vi "OdometrySubscriber.vi"() -> ()   [LabVIEW 2014]
doc: "Reads in the odometry from the Turtlebot"
uses:
  <vilib>/Tufts CEEO ROS for LabVIEW Software/ROS/Code/Console/Servers/ServerSubs/TopicDef.ctl
  <vilib>/Tufts CEEO ROS for LabVIEW Software/ROS/Code/SubVIs/_ROSDirection.ctl
panel:
  out "Odom Error Out":errorcluster
  in  "Update Time (ms)":u32
  in  "Clear Plot":bool
  out "2D Pose":cluster{"x":dbl, "y":dbl}
  out "Position Plot":cluster{"X":dbl, "Y":dbl}[](graph)
  out "Husky EKF Odometry":T1
  in  "Stop Subscribing":bool
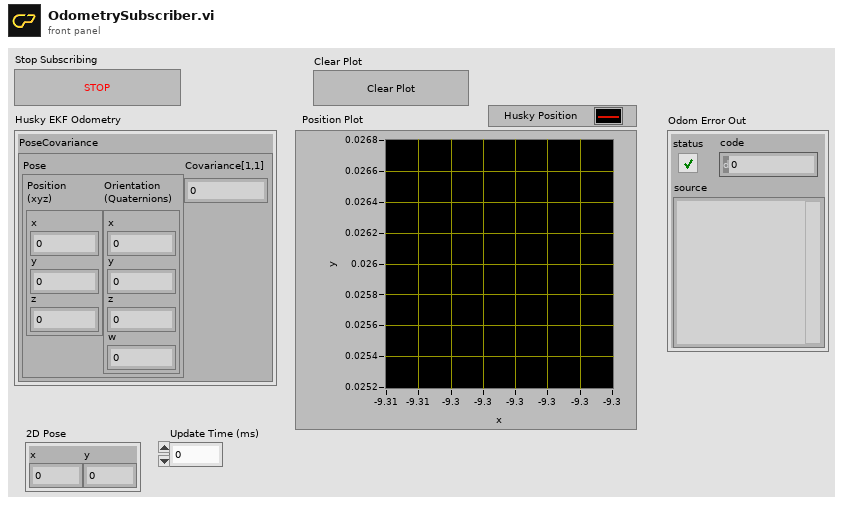
[diagram p1: front panel]
types:
  T1 = cluster{"PoseCovariance":cluster{"Pose":cluster{"Position\n(xyz)":cluster{"x":dbl, "y":dbl, "z":dbl}, "Orientation\n(Quaternions)":cluster{"x":dbl, "y":dbl, "z":dbl, "w":dbl}}, "Covariance[1,1]":dbl}}
  T2 = typedef "TopicDef.ctl" = cluster{"Topic":string, "Type":string, "Action":T3, "Update (ms)":u16, "queue size":u16}
  T3 = typedef "_ROSDirection.ctl" = enum16{"Node", "Publisher", "Subscriber", "ServiceClient", "ServiceProvider"}
  T4 = typedef "_ROSControl.ctl" = cluster{"topic port":u16, "Node":string, "topic":string, "type":string, "node port":u16, "error ":errorcluster, "Direction":T3, "Update (ms)":u16, "FIFO size":u16}
  T5 = cluster{"PoseCovariance":cluster{"Pose":cluster{"Point":cluster{"x":dbl, "y":dbl, "z":dbl}, "Quaternion":cluster{"x":dbl, "y":dbl, "z":dbl, "w":dbl}}, "Covariance":dbl}}
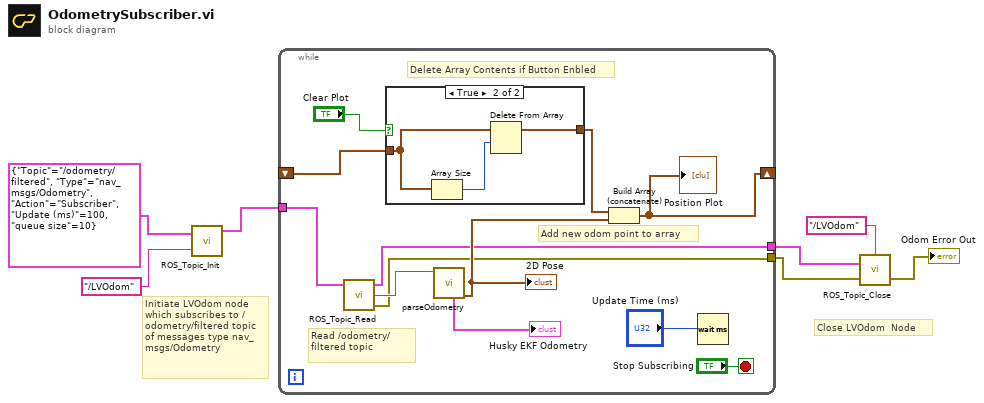
[diagram p0: block diagram]
diagram:
  # "Initiate LVOdom node which subscribes to /odometry/filtered topic of messages type nav_msgs/Odometry"
  # "Close LVOdom  Node"
  n1 = call <vilib>:"ROS_Topic_Init.vi"("Definitions"=T2 {"Topic"="/odometry/filtered", "Type"="nav_msgs/Odometry", "Action"=enum."Subscriber", "Update (ms)"=100, "queue size"=10}, "node"="/LVOdom") -> ("ROS out"=w5:T4)  [unwired: 1 in, 1 out]
  n2 = while {
    shift-right: [w13] -> _
    shift-left: _ -> [w14]
    tunnel: w5 -> [w16]
    tunnel: [w9] -> w2
    tunnel: [w8] -> w1
    stop <- "Stop Subscribing" stop-if-true
    # "Read /odometry/filtered topic"
    # "Add new odom point to array"
    # "Delete Array Contents if Button Enbled"
    n3 = call <vilib>:"ROS_Topic_Read.vi"("ROS in"=w16) -> ("error out"=w8:errorcluster, "Reply"=w18:string, "ROS out"=w9:T4)  [unwired: 2 in]
    n4 = case shown="True" "Clear Plot" {
      tunnel: w14 -> [w20 w21]
      tunnel: [w20 w22] -> w12
      frame False {
      }
      frame True {
        n5 = Array Size(array=w21) -> (size(s)=w23:i32)
        n6 = Delete From Array "Delete From Array"(array=w21, length=w23) -> (array with subset deleted=w22:cluster{"x":dbl, "y":dbl}[])  [unwired: 1 in, 1 out]
      }
    }
    n7 = call "parseOdometry.vi"("msg in"=w18) -> ("Odometry"=→"Husky EKF Odometry":T5, "Pose 2D"=w15:cluster{"x":dbl, "y":dbl})  [unwired: 3 in, 3 out]
    "2D Pose" <- w15
    n8 = Build Array (concatenate)(w12, w15) -> (w13:cluster{"x":dbl, "y":dbl}[])
    "Position Plot" <- w13
    n9 = Wait (ms)(milliseconds to wait="Update Time (ms)") -> ()  [unwired: 1 out]
  }
  n10 = call <vilib>:"ROS_Topic_Close.vi"("error in"=w1, "ROS in"=w2, "node"="/LVOdom") -> ("error out"=→"Odom Error Out":errorcluster)  [unwired: 1 in]
